vi "DLTS - reset impedance (SubVI).vi"(8 "error in (no error)":errorcluster, 11 "Handle in":T1 {"Handle" format="0x%08x"; "Conn" format="0x%08x"}) -> (0 "error out":errorcluster, 3 "Handle out":T1 {"Handle" format="0x%08x"; "Conn" format="0x%08x"})   [LabVIEW 2019]
doc: "Resets impedance analyzers settings after DLTS measurement"
uses:
  <instrlib>/Zurich Instruments LabOne/Public/ziTypeHandle.ctl
  <instrlib>/Zurich Instruments LabOne/Public/Configure/ziSetValueDoubleArray.vi
  <instrlib>/Zurich Instruments LabOne/Zurich Instruments LabOne.lvlib
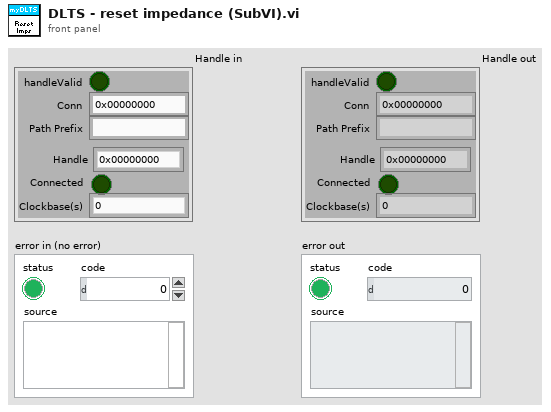
[diagram p1: front panel]
types:
  T1 = typedef "Zurich Instruments LabOne.lvlib/ziTypeHandle.ctl" = cluster{"handleValid":bool, "Conn":u64, "Path Prefix":string, "Handle":u64, "Connected":bool, "Clockbase(s)":dbl}
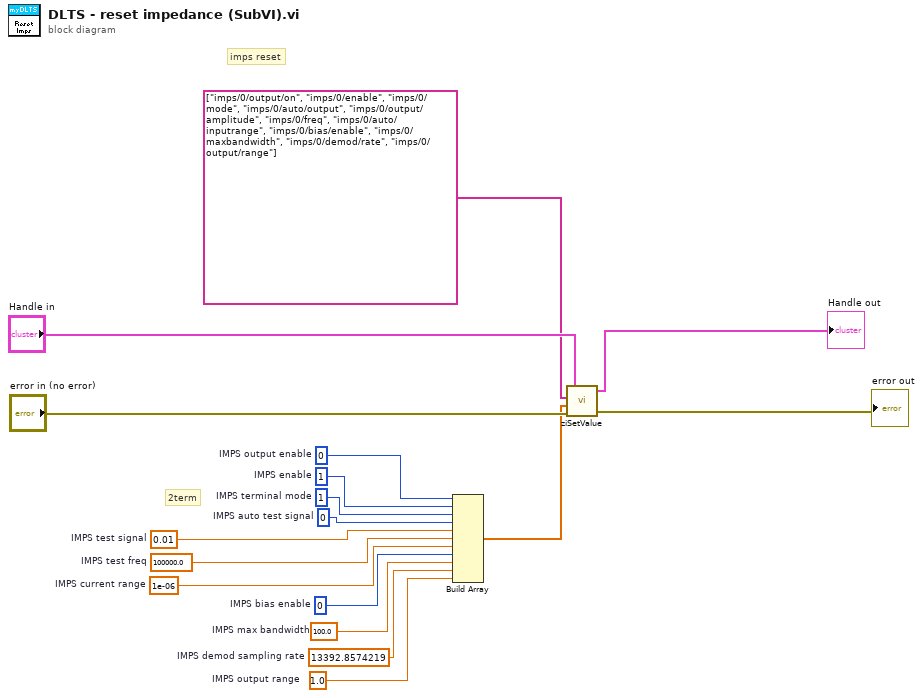
[diagram p0: block diagram]
diagram:
  w11 = 1  # IMPS terminal mode
  w13 = 1.0  # IMPS output range
  w1 = 0  # IMPS output enable
  w12 = 13392.8574219  # IMPS demod sampling rate
  w7 = 100.0  # IMPS max bandwidth
  w6 = 0  # IMPS bias enable
  w5 = 1e-06  # IMPS current range
  w4 = 100000.0  # IMPS test freq
  w3 = 0.01  # IMPS test signal
  w2 = 0  # IMPS auto test signal
  w10 = 1  # IMPS enable
  # "2term"
  # "imps reset"
  n1 = Build Array(w1, w10, w11, w2, w3, w4, w5, w6, w7, w12, w13) -> (w8:dbl[])
  n2 = call-poly <instrlib>:"ziSetValue.vi"("Error In"="error in (no error)", "Values"=w8, "Paths"=string[] ["imps/0/output/on", "imps/0/enable", "imps/0/mode", "imps/0/auto/output", "imps/0/output/amplitude", "imps/0/freq", "imps/0/auto/inputrange", "imps/0/bias/enable", "imps/0/maxbandwidth", "imps/0/demod/rate", "imps/0/output/range"], "Handle In"="Handle in") -> ("Error Out"=→"error out":errorcluster, "Handle Out"=→"Handle out":T1)  [unwired: 1 in]
